vi "GetGetUFastEnabled.vi"(10 "TSRefShot":bool, 11 "Trigger Data":T3) -> (3 "UFast Enabled":bool)   [LabVIEW 2016]
uses:
  Ctrl_Signal.ctl
  Ctrl_Signal_Map.ctl
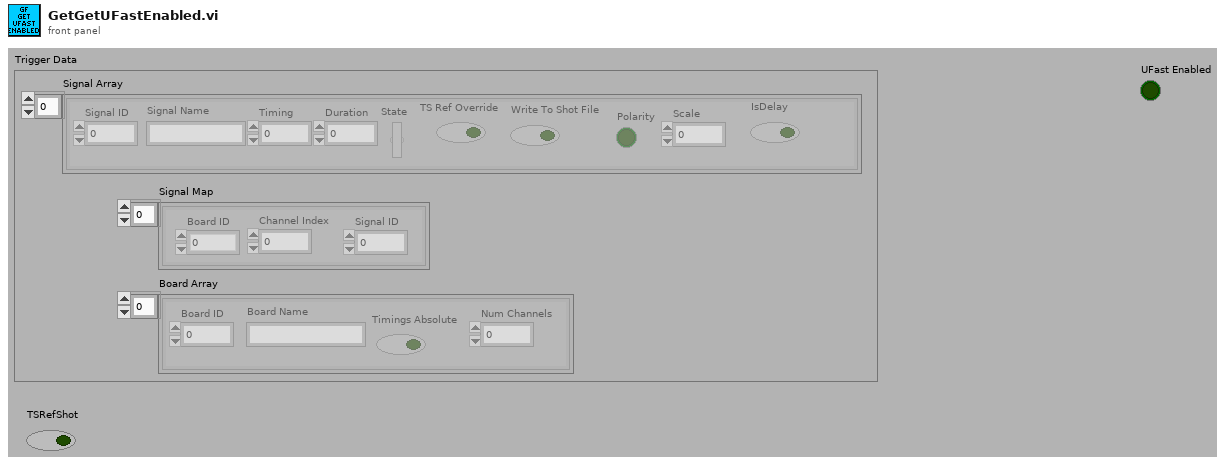
[diagram p1: front panel]
types:
  T1 = typedef "Ctrl_Signal.ctl" = cluster{"Signal Name":string, "Timing":dbl, "Duration":dbl, "State":bool, "TS Ref Override":bool, "Write To Shot File":bool, "Polarity":bool, "Signal ID":dbl, "Scale":dbl, "IsDelay":bool}
  T2 = typedef "Ctrl_Signal_Map.ctl" = cluster{"Channel Index":dbl, "Board ID":dbl, "Signal ID":dbl}
  T3 = cluster{"Signal Array":T1[], "Signal Map":T2[], "Board Array":cluster{"Board ID":dbl, "Board Name":string, "Timings Absolute":bool, "Num Channels":dbl}[]}
  T4 = cluster{"Board ID":dbl, "Board Name":string, "Timings Absolute":bool, "Num Channels":dbl}
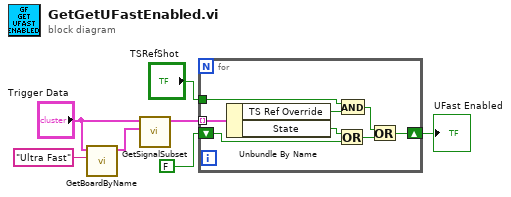
[diagram p0: block diagram]
diagram:
  n1 = call "GetBoardByName.vi"("Board Name"="Ultra Fast", "Trigger Data"="Trigger Data") -> ("Selected Board"=w5:T4)  [unwired: 9 in]
  n2 = call "GetSignalSubset.vi"("Selected Board"=w5, "Trigger Data Input"="Trigger Data") -> ("Signal Subset"=w4:T1[])  [unwired: 9 in]
  n3 = for {
    tunnel: w4 -> [w15] mode=indexing
    shift-right: [w11] -> w2
    shift-left: FALSE -> [w14]
    tunnel: "TSRefShot" -> [w10]
    n4 = Unbundle By Name(w15) -> ("TS Ref Override"=w8:bool, "State"=w9:bool)
    n5 = Or(x=w9, y=w14) -> (x .or. y?=w13:bool)
    n6 = And(x=w10, y=w8) -> (x .and. y?=w12:bool)
    n7 = Or(x=w12, y=w13) -> (x .or. y?=w11:bool)
  }
  "UFast Enabled" <- w2
